vi "Global_Dashboard Controls.vi"() -> ()   [LabVIEW 2017, in "DashBoardCom.lvlib"]
uses:
  DashBoardCom.lvlib
  Shared Code/TypeDefs/Cluster_DashBoard to Rio Controls.ctl
  Shared Code/TypeDefs/ENUM_Auto Select.ctl
panel:
  out "DashboardCom_DB to Rio":T1
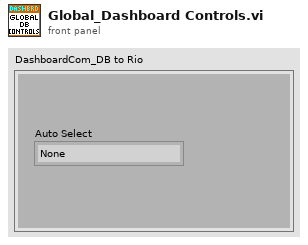
[diagram p1: front panel]
types:
  T1 = typedef "Cluster_DashBoard to Rio Controls.ctl" = cluster{"Auto Select":T2}
  T2 = typedef "ENUM_Auto Select.ctl" = enum16{"None", "Cross Baseline", "Shoot", "Middle Peg", "Right Peg", "Left Peg", "Middle Peg and Shoot", "Side Peg and Shoot", "Dump Hopper and Shoot"}
diagram:
